vi "Initialize Transfer Group.vi"(5 "FIFO Options":T1, 6 "Transfer Group Status":refnum<class "Status Pointer.lvclass">, 7 "id":i32, 8 "error in (no error)":errorcluster, 9 "force inline? (F)":bool, 10 "Transfer Group Buffers":refnum<class "Buffers.lvclass">, 11 "Transfer Group Configuration":T2={"name"="", "direction"=enum."Tx", "cycle timing"={"priority"=0, "decimation"=1, "offset"=0}, "thread index"=255, "settings"=[], "transfers"=[], "timeout behavior"=enum."Increment Late Count", "enable buffer conversion"=FALSE} {"transfers"."channels"."string offset" format="%d bytes"}) -> (0 "error out":errorcluster, 3 "Transfer Group out":refnum<class "Transfer Group.lvclass">)   [LabVIEW 2017, in "DSF Core.lvlib" / "Transfer Group.lvclass"]
uses:
  Transfer Group.lvclass
  Typedefs/DSF Engine Transfer Group Configuration.ctl
  Typedefs/DSF Direction.ctl
  Typedefs/DSF Timing Info.ctl
  Typedefs/DSF Settings Info.ctl
  Typedefs/DSF Engine Transfer Configuration.ctl
  Typedefs/DSF Byte Order.ctl
  Typedefs/DSF Engine Channel Configuration.ctl
  Typedefs/DSF Data Type.ctl
  Typedefs/DSF Timeout Behavior.ctl
  Buffers/Buffers.lvclass
  Typedefs/DSF FIFO Options.ctl
  Status/Status Pointer.lvclass
  Configuration/Required Buffer Size (Transfer).vi
  Transfer/Transfer.lvclass
  Configuration/Configuration Session.lvclass
  DSF Core.lvlib
  Framework/Framework.lvclass
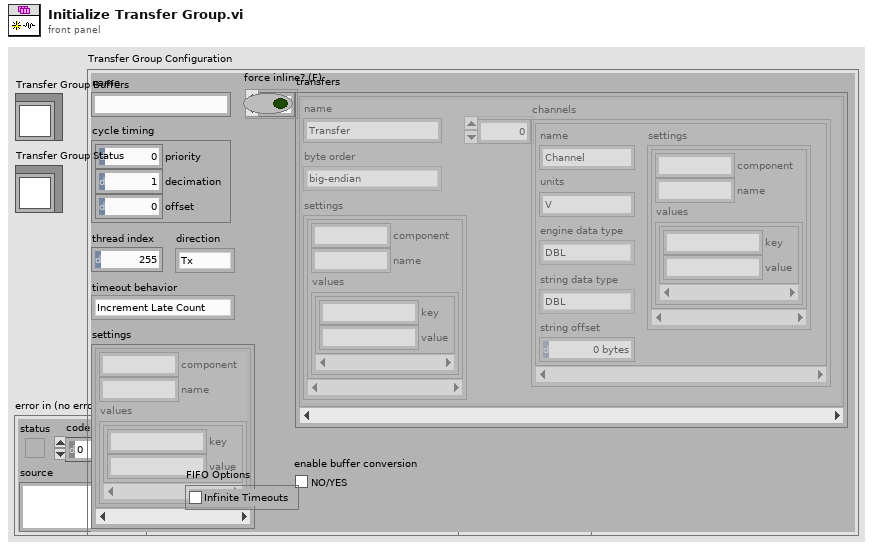
[diagram p1: front panel]
types:
  T1 = typedef "DSF Core.lvlib/Framework.lvclass/DSF FIFO Options.ctl" = cluster{"Infinite Timeouts":bool}
  T2 = typedef "DSF Core.lvlib/DSF Engine Transfer Group Configuration.ctl" = cluster{"name":string, "direction":T3, "cycle timing":T4, "thread index":u8, "settings":T5, "transfers":T6[], "timeout behavior":T10, "enable buffer conversion":bool}
  T3 = typedef "DSF Core.lvlib/DSF Direction.ctl" = enum8{"Tx", "Rx"}
  T4 = typedef "DSF Core.lvlib/DSF Timing Info.ctl" = cluster{"priority":u64, "decimation":u64, "offset":u64}
  T5 = typedef "DSF Core.lvlib/DSF Settings Info.ctl" = cluster{"component":string, "name":string, "values":cluster{"key":string, "value":string}[]}[]
  T6 = typedef "DSF Core.lvlib/DSF Engine Transfer Configuration.ctl" = cluster{"name":string, "byte order":T7, "settings":T5, "channels":T8[]}
  T7 = typedef "DSF Core.lvlib/DSF Byte Order.ctl" = enum8{"big-endian", "little-endian"}
  T8 = typedef "DSF Core.lvlib/DSF Engine Channel Configuration.ctl" = cluster{"string offset":u64, "name":string, "units":string, "engine data type":T9, "string data type":T9, "settings":T5}
  T9 = typedef "DSF Core.lvlib/DSF Data Type.ctl" = enum8{"Bool", "SGL", "DBL", "I8", "I16", "I32", "I64", "U8", "U16", "U32", "U64"}
  T10 = typedef "DSF Core.lvlib/DSF Timeout Behavior.ctl" = enum8{"Increment Late Count", "Throw Error"}
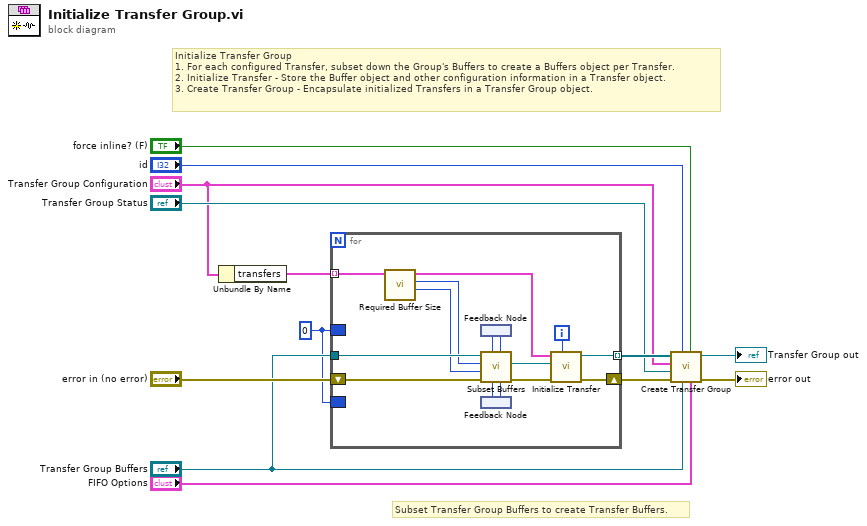
[diagram p0: block diagram]
diagram:
  w7 = u64 0 ("inline buffer size")
  # "Initialize Transfer Group\n1. For each configured Transfer, subset down the Group's Buffers to create a Buffers object per Transfer.\n2. Initialize Transfer - Store the Buffer object and other configuration information in a Transfer object.\n3. Create Transfer Group - Encapsulate initialized Transfers in a Transfer Group object."
  # "Subset Transfer Group Buffers to create Transfer Buffers."
  n1 = Unbundle By Name("Transfer Group Configuration") -> ("transfers"=w12:T6[])
  n2 = for {
    tunnel: w12 -> [w25] mode=indexing
    tunnel: [w28] -> w10 mode=indexing
    shift-right: [w27] -> w11
    shift-left: "error in (no error)" -> [w24]
    border: w7 -> [_]
    border: w7 -> [_]
    tunnel: "Transfer Group Buffers" -> [w23]
    i -> [w26]
    n3 = call-poly "Required Buffer Size.vi"("Transfer Configuration in"=w25) -> ("engine buffer size"=w15:u64, "string buffer size"=w16:u64, "Transfer Configuration out"=w14:T6)  [unwired: 7 in, 1 out]
    n4 = feedback #1() -> (w20:u64)
    n5 = feedback #2() -> (w22:u64)
    n6 = call "Subset Buffers.vi"("inline buffer offset"=w22, "string buffer offset"=w20, "error in (no error)"=w24, "inline buffer size"=w15, "string buffer size"=w16, "Buffers in"=w23) -> ("error out"=w18:errorcluster, "subset Buffers"=w17:refnum<class "Buffers.lvclass">, "inline buffer offset +size"=w21:u64, "string buffer offset + size"=w19:u64)  [unwired: 1 in, 1 out]
    n7 = feedback-in #1(w19) -> ()
    n8 = feedback-in #2(w21) -> ()
    n9 = call "Initialize Transfer.vi"("id"=w26, "error in (no error)"=w18, "Buffers"=w17, "Transfer Configuration"=w14) -> ("error out"=w27:errorcluster, "Transfer out"=w28:refnum<class "Transfer.lvclass">)  [unwired: 6 in]
  }
  n10 = call "Create Transfer Group.vi"("FIFO Options"="FIFO Options", "force inline? (F)"="force inline? (F)", "Buffers"="Transfer Group Buffers", "id"="id", "error in (no error)"=w11, "Transfer Group Status"="Transfer Group Status", "Transfer Group configuration"="Transfer Group Configuration", "Transfers"=w10) -> ("error out"=→"error out":errorcluster, "Transfer Group out"=→"Transfer Group out":refnum<class "Transfer Group.lvclass">)  [unwired: 2 in]
